vi "Write TDMS Data - Simple Example.vi"   [LabVIEW 2014]
types:
  T1 = enum16{"open", "open or create", "create or replace", "create", "open (read-only)"}
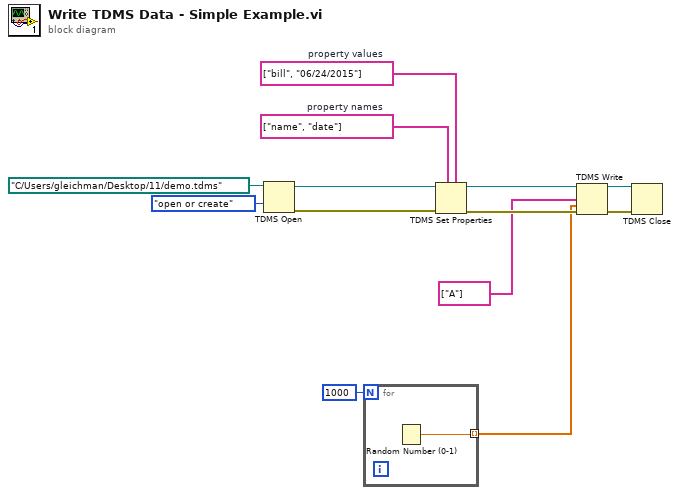
[diagram p0: block diagram]
diagram:
  w10 = string[] ["bill", "06/24/2015"]  # property values
  w11 = string[] ["name", "date"]  # property names
  n1 = TDMS Open(10:T1."open or create" ("operation (0:open)"), 11:path "C:/Users/gleichman/Desktop/11/demo.tdms" ("file path")) -> (0:w13:errorcluster, 3:w12:refnum<k34>)  [unwired: 5 in]
  n2 = for {
    N: 1000 -> [_]
    tunnel: [w14] -> w6 mode=indexing
    n3 = Random Number (0-1)() -> (number: 0 to 1=w14:dbl)
  }
  n4 = TDMS Set Properties(5:w10, 7:w11, 8:w13, 11:w12) -> (0:w9:errorcluster, 3:w8:refnum<k34>)  [unwired: 2 in, 2 out]
  n5 = TDMS Write(0:w8, 7:string[] ["A"] ("channel name(s) in (Untitled)"), 9:w6, 11:w9) -> (4:w3:refnum<k34>, 15:w4:errorcluster)  [unwired: 2 in, 2 out]
  n6 = TDMS Close(8:w4, 11:w3) -> ()  [unwired: 2 out]
